vi "Example Callback.vi"() -> ()   [LabVIEW 2013]
uses:
  C:/tf/play/labview/Tinkerforge.dll
  Tinkerforge.dll
panel:
  out "altitude (m)":sgl format="%#_13g"
  in  "stop":bool
  out "air pressure (mbar)":sgl format="%#_13g"
  in  "uid":string="jmQ"
  in  "port":i32=4223
  in  "host":string="localhost"
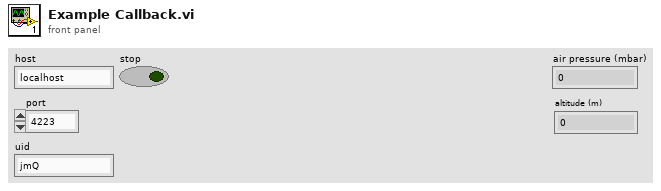
[diagram p1: front panel]
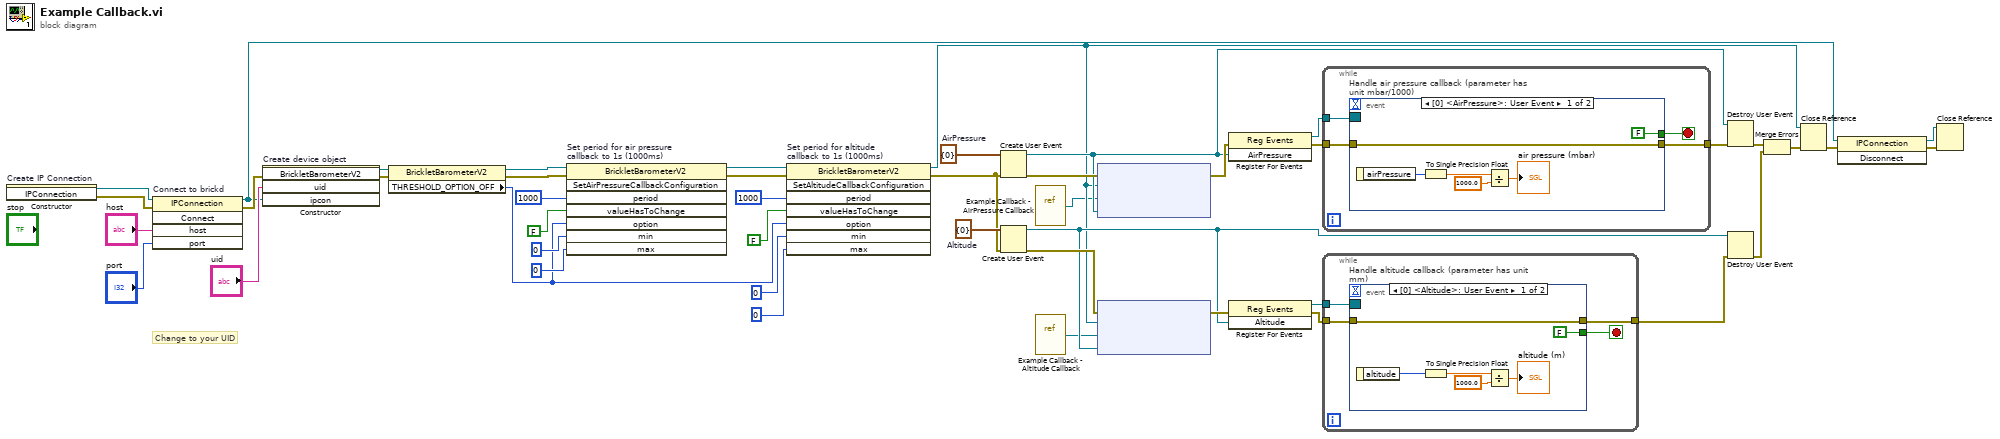
[diagram p0: block diagram]
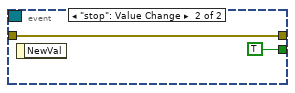
[diagram p2: hidden frame]
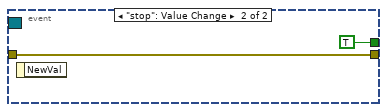
[diagram p3: hidden frame]
diagram:
  w22 = cluster{"altitude":i32} {"altitude"=0}  # Altitude
  w31 = cluster{"airPressure":i32} {"airPressure"=0}  # AirPressure
  # "Change to your UID"
  n1 = constructor on="Create IP Connection" class="IPConnection"() -> (reference out=w46:refnum<k24>, error out=w12:errorcluster)  [unwired: 3 in, 1 out]
  n2 = invoke on="Connect to brickd" class="IPConnection" method="Connect"(reference=w46, error in=w12, "host"="host", "port"="port") -> (reference out=w39:refnum<k24>, error out=w42:errorcluster)  [unwired: 1 in, 3 out]
  n3 = constructor on="Create device object" class="BrickletBarometerV2"(error in=w42, "uid"="uid", "ipcon"=w39) -> (reference out=w2:refnum<k24>, error out=w5:errorcluster)  [unwired: 2 in, 3 out]
  n4 = property class="BrickletBarometerV2"(reference=w2, error in=w5) -> (reference out=w3:refnum<k24>, error out=w4:errorcluster, "THRESHOLD_OPTION_OFF"=w1:u16)
  n5 = invoke on="Set period for air pressure\ncallback to 1s (1000ms)" class="BrickletBarometerV2" method="SetAirPressureCallbackConfiguration"(reference=w3, error in=w4, "period"=i64 1000, "valueHasToChange"=FALSE, "option"=w1, "min"=0, "max"=0) -> (reference out=w15:refnum<k24>, error out=w16:errorcluster)  [unwired: 1 in, 6 out]
  n6 = invoke on="Set period for altitude\ncallback to 1s (1000ms)" class="BrickletBarometerV2" method="SetAltitudeCallbackConfiguration"(reference=w15, error in=w16, "period"=i64 1000, "valueHasToChange"=FALSE, "option"=w1, "min"=0, "max"=0) -> (reference out=w23:refnum<k24>, error out=w21:errorcluster)  [unwired: 1 in, 6 out]
  n7 = Create User Event(user event datatype=w31, error in=w21) -> (user event=w32:refnum<user-event>, error out=w37:errorcluster)
  n8 = Create User Event(user event datatype=w22, error in=w21) -> (user event=w24:refnum<user-event>, error out=w29:errorcluster)
  n9 = vi-ref "Example Callback - AirPressure Callback.vi"() -> ("vi reference"=w14:refnum<vi>)
  n10 = vi-ref "Example Callback - Altitude Callback.vi"() -> ("vi reference"=w13:refnum<vi>)
  n11 = node ("Register Event Callback")(w37, w23, w14, w32) -> (w36:errorcluster)  [unwired: 1 in, 1 out]
  n12 = node ("Register Event Callback")(w29, w23, w13, w24) -> (w28:errorcluster)  [unwired: 1 in, 1 out]
  n13 = register-events(error in=w36, w32) -> (reference out=w35:refnum<event-registration>, error out=w33:errorcluster)  [unwired: 1 in]
  n14 = register-events(error in=w28, w24) -> (reference out=w27:refnum<event-registration>, error out=w25:errorcluster)  [unwired: 1 in]
  n15 = while {
    tunnel: w35 -> [w50]
    tunnel: [w49] -> w34
    tunnel: w33 -> [w48]
    stop <- w47 stop-if-true
    n16 = event "Handle air pressure callback (parameter has unit mbar/1000)" shown="[0] <AirPressure>: User Event" {
      selector: w50 -> [_ _]
      dyn-events: _ -> [_ _]
      timeout: _ -> [_ _]
      tunnel: [w53 w57] -> w49
      tunnel: w48 -> [w53 w57]
      tunnel: [FALSE TRUE] -> w47
      event User Event {
        n17 = event-data() -> ("airPressure"=w54:i32)  [unwired: 1 in]
        n18 = To Single Precision Float(number=w54) -> (single precision float=w55:sgl)
        n19 = Divide(x=w55, y=sgl 1000.0) -> (x/y=→"air pressure (mbar)":sgl)
      }
      event "stop": Value Change {
        n20 = event-data() -> ()  [unwired: 1 in, 1 out]
      }
    }
  }
  n21 = while {
    tunnel: w27 -> [w62]
    tunnel: [w61] -> w26
    tunnel: w25 -> [w60]
    stop <- w59 stop-if-true
    n22 = event "Handle altitude callback (parameter has unit mm)" shown="[0] <Altitude>: User Event" {
      selector: w62 -> [_ _]
      dyn-events: _ -> [_ _]
      timeout: _ -> [_ _]
      tunnel: [w65 w69] -> w61
      tunnel: w60 -> [w65 w69]
      tunnel: [FALSE TRUE] -> w59
      event User Event {
        n23 = event-data() -> ("altitude"=w66:i32)  [unwired: 1 in]
        n24 = To Single Precision Float(number=w66) -> (single precision float=w67:sgl)
        n25 = Divide(x=w67, y=sgl 1000.0) -> (x/y=→"altitude (m)":sgl)
      }
      event "stop": Value Change {
        n26 = event-data() -> ()  [unwired: 1 in, 1 out]
      }
    }
  }
  n27 = Destroy User Event(user event=w32, error in=w34) -> (error out=w19:errorcluster)
  n28 = Destroy User Event(user event=w24, error in=w26) -> (error out=w20:errorcluster)
  n29 = Merge Errors(w19, w20) -> (w18:errorcluster)
  n30 = Close Reference(reference=w23, error in (no error)=w18) -> (error out=w41:errorcluster)
  n31 = invoke class="IPConnection" method="Disconnect"(reference=w39, error in=w41) -> (reference out=w38:refnum<k24>, error out=w40:errorcluster)  [unwired: 1 in, 1 out]
  n32 = Close Reference(reference=w38, error in (no error)=w40) -> ()  [unwired: 1 out]
